vi "Configure Reference Oscillator.vi"(8 "error in (no error)":errorcluster, 10 "Reference Mode":enum16{"Internal", "External"}(ring), 11 "SigGen-SMBV in":refnum<class "VSG-SMBV.lvclass">) -> (0 "error out":errorcluster, 3 "SigGen-SMBV out":refnum<class "VSG-SMBV.lvclass">)   [LabVIEW 2020, in "VSG-SMBV.lvclass"]
uses:
  VSG-SMBV.lvclass
  C:/Sandbox/RF Bench/Source Code/WiSpry Test Framework/Instruments/Vector Signal Generator/Vector Signal Generator.lvclass
  C:/Sandbox/RF Bench/Source Code/WiSpry Test Framework/Instruments/Instrument.lvclass
  Vector Signal Generator.lvclass/Vector Signal Generator.ctl
  Instrument.lvclass/Instrument.ctl
  Instrument.lvclass
  Vector Signal Generator.lvclass
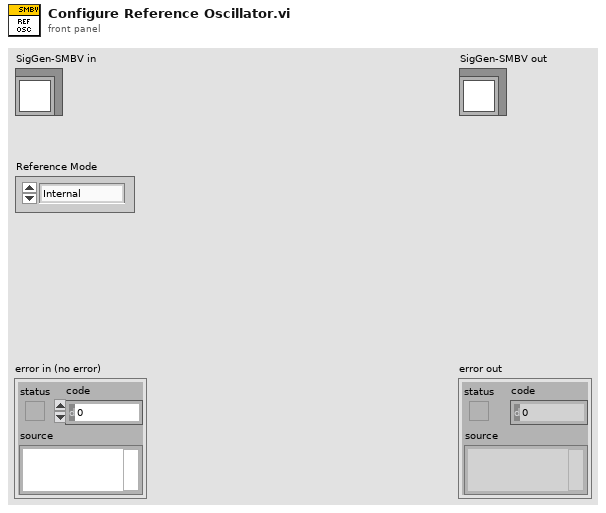
[diagram p1: front panel]
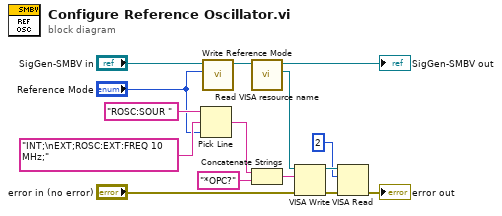
[diagram p0: block diagram]
diagram:
  n1 = Pick Line(string ("")="ROSC:SOUR ", multi-line string="INT;\nEXT;ROSC:EXT:FREQ 10 MHz;", line index="Reference Mode") -> (output string=w11:string)
  n2 = call "Write Reference Mode.vi"("Reference Mode"="Reference Mode", "Signal Generator in"="SigGen-SMBV in") -> ("Signal Generator out"=w9:refnum<class "VSG-SMBV.lvclass">)  [unwired: 9 in]
  n3 = call "Read VISA resource name.vi"("Instrument in"=w9) -> ("VISA resource name"=w7:refnum<visa-resource-name>, "Instrument out"=→"SigGen-SMBV out":refnum<class "VSG-SMBV.lvclass">)  [unwired: 9 in]
  n4 = Concatenate Strings(w11, "*OPC?" ("string")) -> (w6:string)
  n5 = VISA Write(VISA resource name=w7, write buffer=w6, error in (no error)="error in (no error)") -> (VISA resource name out=w3:refnum<visa-resource-name>, error out=w4:errorcluster)  [unwired: 1 out]
  n6 = VISA Read(VISA resource name=w3, byte count=u32 2, error in (no error)=w4) -> (error out=→"error out":errorcluster)  [unwired: 3 out]
